vi "Get Debug Mode.vi"(8 "error in (no error)":errorcluster, 11 "SMO":refnum<class "SMO.lvclass">) -> (0 "error out":errorcluster, 2 "Behavior":T1, 3 "SMO out":refnum<class "SMO.lvclass">)   [LabVIEW 2019, in "SMO Debug.lvlib"]
uses:
  SMO Debug.lvlib
  <vilib>/JKI/JKI SMO/SMO/SMO.lvclass
  Attribute.Debug/DebugBehavior.ctl
  Attribute.Debug/Attribute.Debug.lvclass/Attribute.Debug.ctl
  SMO.Mediator.lvclass
  Attribute.Debug/Attribute.Debug.lvclass
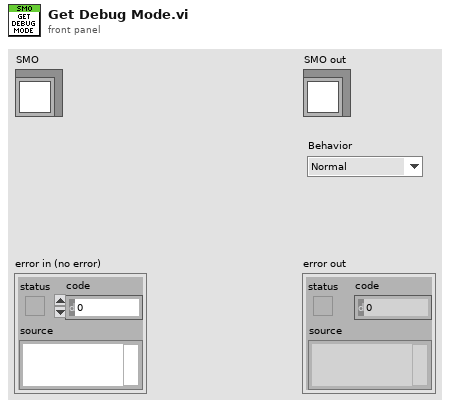
[diagram p1: front panel]
types:
  T1 = typedef "SMO Debug.lvlib/Attribute.Debug.lvclass/DebugBehavior.ctl" = enum16{"Normal", "Debug"}
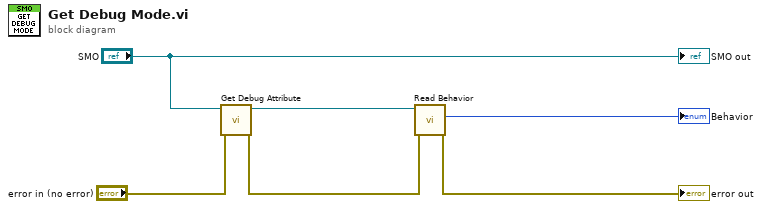
[diagram p0: block diagram]
diagram:
  n1 = call "Get Debug Attribute.vi"("error in (no error)"="error in (no error)", "SMO"="SMO") -> ("error out"=w2:errorcluster, "Attribute.Debug"=w4:refnum<class "Attribute.Debug.lvclass">)  [unwired: 8 in]
  n2 = call "Read Behavior.vi"("error in (no error)"=w2, "Attribute.StartupBehavior in"=w4) -> ("error out"=→"error out":errorcluster, "Behavior"=→"Behavior":T1)  [unwired: 7 in, 1 out]
  "SMO out" <- "SMO"
